vi "service_error_parse.vi"(3 "error in (no error)":errorcluster, 5 "Reply":string="\u0000\u0000\u0000\u0000\u0000") -> (0 "error out":errorcluster, 1 "OK?":bool, 2 "Error Code":i32)   [LabVIEW 2012]
doc: "Parses a message into a service error"
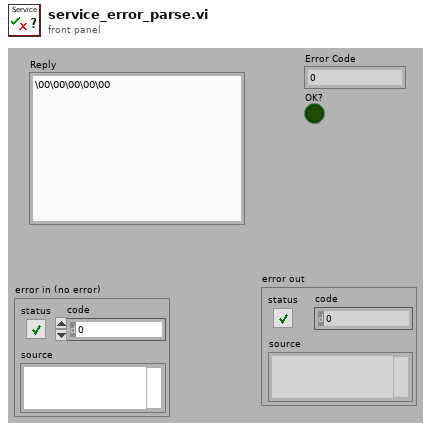
[diagram p1: front panel]
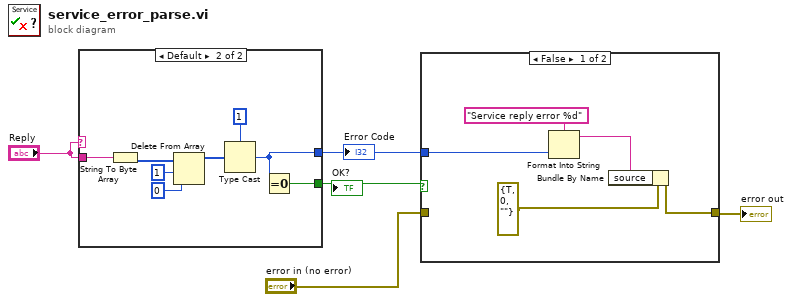
[diagram p0: block diagram]
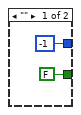
[diagram p3: hidden frame]
diagram:
  n1 = case shown="Default" "Reply" {
    tunnel: "Reply" -> [_ w15]
    tunnel: [-1 ("length") w9] -> w1
    tunnel: [FALSE w8] -> w4
    frame "" {
    }
    frame Default {
      n2 = String To Byte Array(string=w15) -> (unsigned byte array=w14:u8[])
      n3 = Delete From Array(array=w14, length=1, index=0) -> (array with subset deleted=w11:u8[])  [unwired: 1 out]
      n4 = Type Cast(type=1 ("length"), x=w11) -> (*(type *) &x=w9:i32)
      n5 = Equal To 0?(x=w9) -> (x = 0?=w8:bool)
    }
  }
  "Error Code" <- w1
  "OK?" <- w4
  n6 = case shown="False" w4 {
    tunnel: [w17 w21] -> w2
    tunnel: "error in (no error)" -> [_ w21]
    tunnel: w1 -> [w19 _]
    frame False {
      n7 = Format Into String(format string="Service reply error %d" ("source"), w19) -> (resulting string=w16:string)  [unwired: 2 in, 1 out]
      n8 = Bundle By Name(cluster=errorcluster {"status"=TRUE, "code"=0, "source"=""} ("error in (no error)"), "source"=w16) -> (w17:errorcluster)
    }
    frame True {
    }
  }
  "error out" <- w2
